vi "Origin_Export.vi"(5 "String 3":string, 6 "error in (no error)":errorcluster, 7 "Array":string[][](array[string]), 8 "String 2":string, 9 "String":string, 10 "Origin.IOApplication":refnum<k7>, 11 "Array 2":string[](array[string])) -> (0 "reference out":refnum<k7>, 1 "error out":errorcluster, 3 "Origin.Worksheet":refnum<k7>)   [LabVIEW 2011]
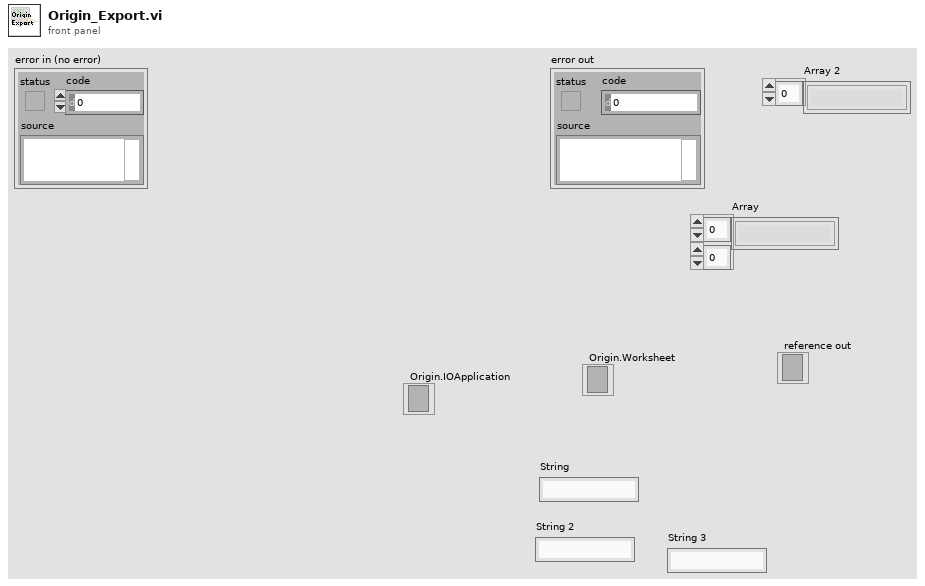
[diagram p1: front panel]
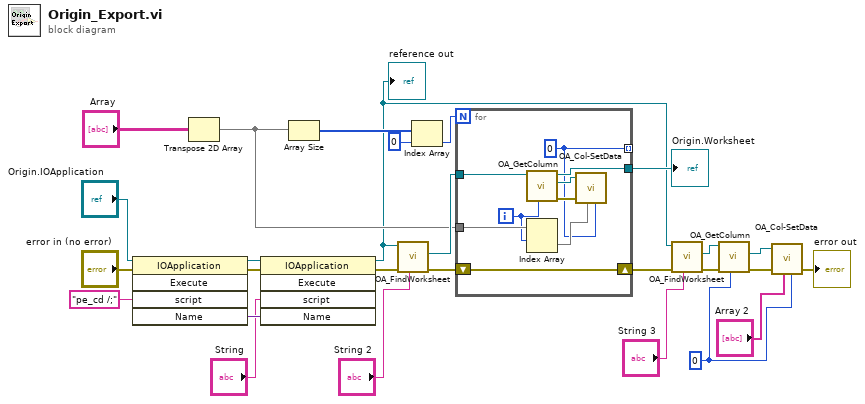
[diagram p0: block diagram]
diagram:
  w4 = 0
  n1 = invoke class="IOApplication" method="Execute"(reference="Origin.IOApplication", error in="error in (no error)", "script"="pe_cd /;") -> (reference out=w26:refnum<k7>, error out=w25:errorcluster, "Name"=w24:variant)  [unwired: 2 in, 2 out]
  n2 = Transpose 2D Array(2D array="Array") -> (transposed array=w15:string[][])
  n3 = invoke class="IOApplication" method="Execute"(reference=w26, error in=w25, "script"="String", "Name"=w24) -> (reference out=w11:refnum<k7>, error out=w10:errorcluster)  [unwired: 1 in, 3 out]
  "reference out" <- w11
  n4 = Array Size(array=w15) -> (size(s)=w21:i32[])
  n5 = call <userlib>:"OA_FindWorksheet.vi"("Name"="String 2", "error in (no error)"=w10, "Origin.IOApplication"=w11) -> ("error out"=w22:errorcluster, "Origin.Worksheet"=w23:refnum<k7>)  [unwired: 6 in, 1 out]
  n6 = Index Array(array=w21, index=0) -> (element=w20:i32)
  n7 = for {
    N: w20 -> [_]
    tunnel: w23 -> [w36]
    tunnel: w15 -> [w35]
    tunnel: [w34] -> w16
    shift-right: [w30] -> w8
    shift-left: w22 -> [w30]
    tunnel: [w28] -> _ mode=indexing
    i -> [w29]
    w28 = 0
    n8 = call <userlib>:"OA_GetColumn.vi"("Column Name/Index"=w29, "Origin.Worksheet"=w36) -> ("error out"=w32:errorcluster, "Origin.Column"=w33:refnum<k7>, "Origin.Worksheet"=w34:refnum<k7>)  [unwired: 7 in]
    n9 = Index Array(array=w35, index (row)=w29) -> (element=w31:string[])  [unwired: 1 in]
    n10 = call <userlib>:"OA_Col-SetData.vi"("Origin.Column"=w33, "error in (no error)"=w32, "data"=w31, "nOffset"=w28) -> ()  [unwired: 3 in, 3 out]
  }
  "Origin.Worksheet" <- w16
  n11 = call <userlib>:"OA_FindWorksheet.vi"("Name"="String 3", "error in (no error)"=w8, "Origin.IOApplication"=w11) -> ("error out"=w3:errorcluster, "Origin.Worksheet"=w7:refnum<k7>)  [unwired: 6 in, 1 out]
  n12 = call <userlib>:"OA_GetColumn.vi"("Column Name/Index"=w4, "error in (no error)"=w3, "Origin.Worksheet"=w7) -> ("error out"=w2:errorcluster, "Origin.Column"=w6:refnum<k7>)  [unwired: 6 in, 1 out]
  n13 = call <userlib>:"OA_Col-SetData.vi"("Origin.Column"=w6, "error in (no error)"=w2, "data"="Array 2", "nOffset"=w4) -> ("error out"=→"error out":errorcluster)  [unwired: 3 in, 2 out]
